vi "estructura_casos_enum.vi"() -> ()   [LabVIEW 2020]
panel:
  in  "OPERACIONES":T1(ring)
  out "RESULTADO":dbl
  in  "NUM2":dbl
  in  "NUM1":dbl
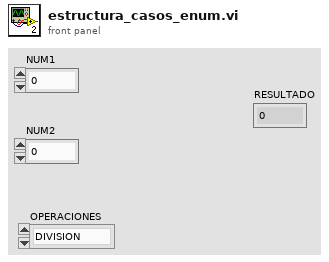
[diagram p1: front panel]
types:
  T1 = enum16{"DIVISION", "MULTIPLICACION", "RESTA", "SUMA"}
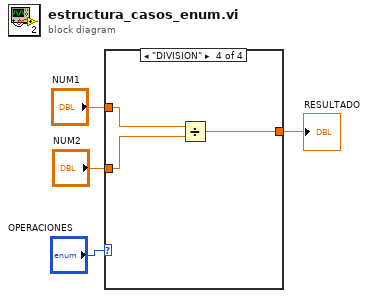
[diagram p0: block diagram]
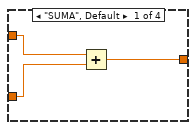
[diagram p2: hidden frame]
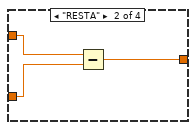
[diagram p3: hidden frame]
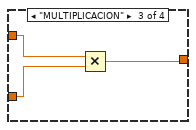
[diagram p4: hidden frame]
diagram:
  n1 = case shown="\"DIVISION\"" "OPERACIONES" {
    tunnel: "NUM1" -> [w7 w10 w13 w16]
    tunnel: "NUM2" -> [w6 w9 w12 w15]
    tunnel: [w5 w8 w11 w14] -> w1
    frame "SUMA", Default {
      n2 = Add(x=w7, y=w6) -> (x+y=w5:dbl)
    }
    frame "RESTA" {
      n3 = Subtract(x=w10, y=w9) -> (x-y=w8:dbl)
    }
    frame "MULTIPLICACION" {
      n4 = Multiply(x=w13, y=w12) -> (x*y=w11:dbl)
    }
    frame "DIVISION" {
      n5 = Divide(x=w16, y=w15) -> (x/y=w14:dbl)
    }
  }
  "RESULTADO" <- w1
